vi "RateLimit.vi"(10 "slew rate":dbl=1.0, 11 "input":dbl) -> (3 "output":dbl)   [LabVIEW 2019]
uses:
  <vilib>/Simulation/Implementation/Shared/SIMSCR Execution Mode.ctl
  <vilib>/Simulation/Scripting/Companion Diagram/SimConfigNode/SimParams.ctl
  <vilib>/Simulation/Scripting/Companion Diagram/SimConfigNode/_simSolvers.ctl
  <vilib>/Simulation/Param Hierarchy/Typedefs/SIMPH Param Control Actions.ctl
  <vilib>/Simulation/Implementation/Shared/NILVSim_ParamChanged.vi
  <vilib>/Simulation/Implementation/Shared/NILVSIM_BeginStep.vi
  <vilib>/Simulation/Nonlinear/Implementation/NILVSim RateLimiter.llb/SIM RateLimiter (scalar).vi
  <vilib>/Simulation/Implementation/Shared/NILVSim_Manager.vi
  <vilib>/Utility/error.llb/Clear Errors.vi
  <vilib>/Simulation/Implementation/Shared/NILVSim_FinalizeModel.vi
  <vilib>/Simulation/Implementation/Shared/SIM Unbundle Sim Info.vi
  <vilib>/Simulation/Implementation/Shared/SIMSH Read Queue.vi
  <vilib>/Simulation/Implementation/Shared/NILVSim_Initialize.vi
  <vilib>/Simulation/Utility/Implementation/NILVSim Get Time and IsAcceptedStep.vi
  <vilib>/Simulation/Implementation/Shared/NILVSim_GetModelError.vi
  <vilib>/Simulation/Implementation/Shared/SIM SimErrorHandler.vi
  <vilib>/Simulation/Implementation/Shared/SIM Bundle Sim Info.vi
  <vilib>/Simulation/Scripting/Companion Diagram/SimConfigNode/SimDog.xnode
  <vilib>/Simulation/Implementation/XNodeFramework/SimXNode/SimX.xnode
  <vilib>/Simulation/Implementation/Shared/NI_SIM_Implementation.lvlib
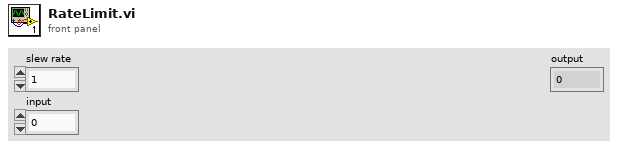
[diagram p1: front panel]
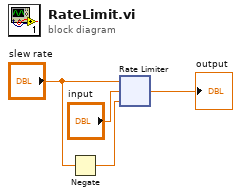
[diagram p0: block diagram]
diagram:
  n1 = Negate(x="slew rate") -> (-x=w2:dbl)
  n2 = xnode "Rate Limiter"("positive slew rate"="slew rate", "input"="input", "negative slew rate"=w2) -> ("output"=→"output":dbl)  [unwired: 2 in]
